vi "Plotter.vi"(1 "3rd":string[](array[string]), 2 "2nd":string[](array[string])) -> (0 "Desired Indicies":i32[](array[numeric]))   [LabVIEW 2010]
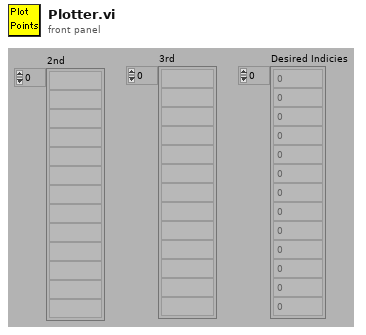
[diagram p1: front panel]
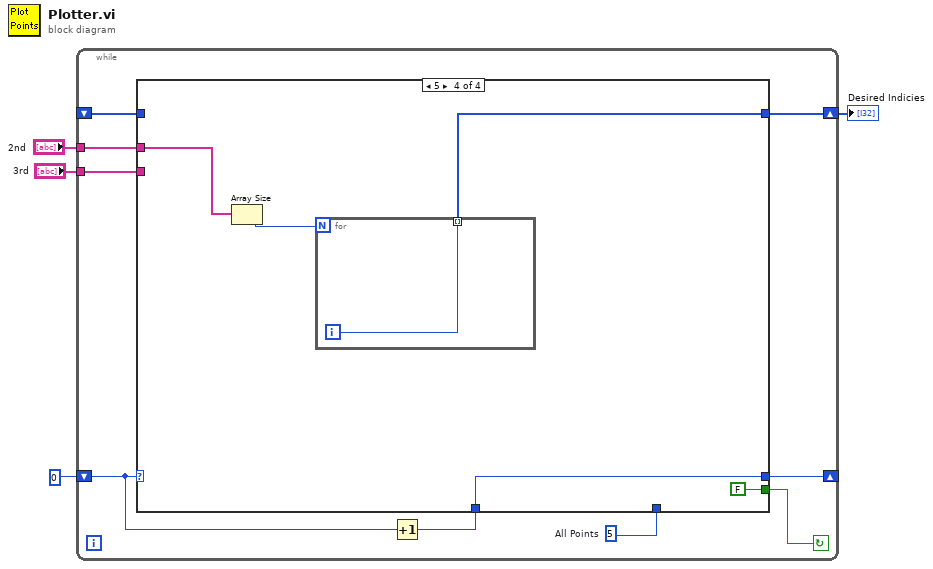
[diagram p0: block diagram]
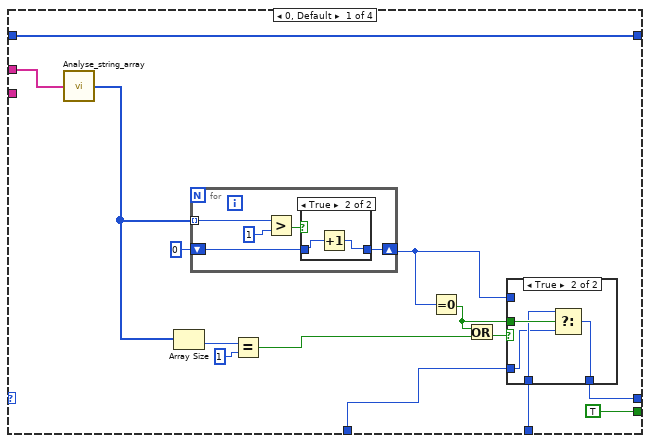
[diagram p2: hidden frame]
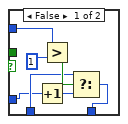
[diagram p3: hidden frame]
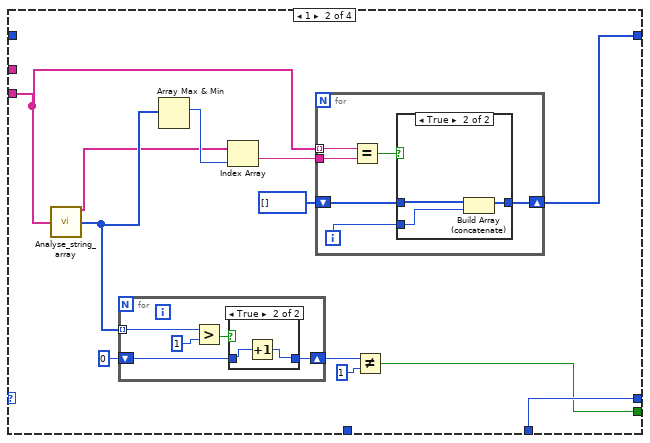
[diagram p5: hidden frame]
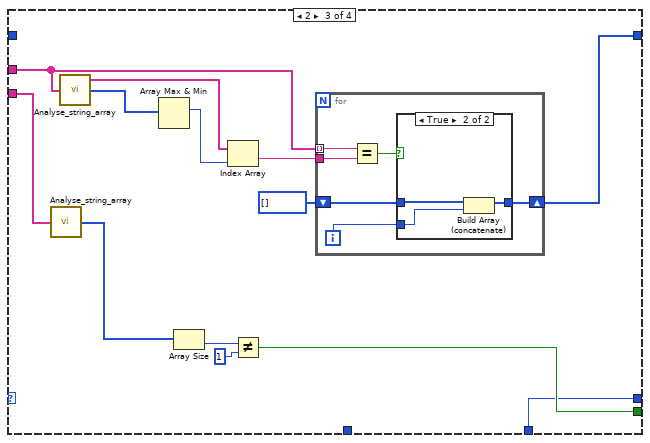
[diagram p8: hidden frame]
diagram:
  n1 = while {
    shift-left: _ -> [w5]
    shift-right: [w7] -> w1
    tunnel: "3rd" -> [w8]
    tunnel: "2nd" -> [w9]
    shift-left: 0 -> [w12]
    shift-right: [w10] -> _
    stop <- w13 continue-if-true
    w6 = 5  # All Points
    n2 = Increment(x=w12) -> (x+1=w11:i32)
    n3 = case shown="5" w12 {
      tunnel: [TRUE w50 w87 FALSE] -> w13
      tunnel: w11 -> [w18 _ _ w100]
      tunnel: [w19 w58 w86 w100] -> w10
      tunnel: w9 -> [w26 _ w79 w104]
      tunnel: w8 -> [_ w47 w80 _]
      tunnel: [w15 w54 w82 w102] -> w7
      tunnel: w6 -> [w16 w58 w86 _]
      tunnel: w5 -> [w15 _ _ _]
      frame 0, Default {
        n4 = call "Analyse_string_array.vi"("String array"=w26) -> ("Frequency"=w24:i32[])  [unwired: 1 in, 1 out]
        n5 = Array Size(array=w24) -> (size(s)=w22:i32)
        n6 = for {
          tunnel: w24 -> [w43] mode=indexing
          shift-right: [w40] -> w17
          shift-left: 0 -> [w39]
          n7 = Greater?(x=w43, y=1) -> (0:w41:bool)
          n8 = case shown="True" w41 {
            tunnel: [w44 w45] -> w40
            tunnel: w39 -> [w44 w46]
            frame False {
            }
            frame True {
              n9 = Increment(x=w46) -> (x+1=w45:i32)
            }
          }
        }
        n10 = Equal?(x=w22, y=1) -> (x = y?=w21:bool)
        n11 = Equal To 0?(x=w17) -> (x = 0?=w14:bool)
        n12 = Or(x=w14, y=w21) -> (x .or. y?=w20:bool)
        n13 = case shown="True" w20 {
          tunnel: [w28 w35] -> w19
          tunnel: w18 -> [w30 w36]
          tunnel: w17 -> [w34 _]
          tunnel: w16 -> [w31 w37]
          tunnel: w14 -> [_ w38]
          frame False {
            n14 = Increment(x=w30) -> (x+1=w29:i32)
            n15 = Greater?(x=w34, y=1) -> (0:w32:bool)
            n16 = Select(t=w31, s=w32, f=w29) -> (s? t:f=w28:i32)
          }
          frame True {
            n17 = Select(t=w37, s=w38, f=w36) -> (s? t:f=w35:i32)
          }
        }
      }
      frame 1 {
        n18 = call "Analyse_string_array.vi"("String array"=w47) -> ("Unique strings"=w48:string[], "Frequency"=w49:i32[])  [unwired: 1 in]
        n19 = for {
          tunnel: w49 -> [w63] mode=indexing
          shift-right: [w60] -> w51
          shift-left: 0 -> [w59]
          n20 = Greater?(x=w63, y=1) -> (0:w61:bool)
          n21 = case shown="True" w61 {
            tunnel: [w64 w65] -> w60
            tunnel: w59 -> [w64 w66]
            frame False {
            }
            frame True {
              n22 = Increment(x=w66) -> (x+1=w65:i32)
            }
          }
        }
        n23 = Array Max & Min(array=w49) -> (max index (indices)=w57:i32)  [unwired: 3 out]
        n24 = Index Array(array=w48, index=w57) -> (element=w56:string)
        n25 = for {
          shift-right: [w68] -> w54
          shift-left: i32[] [] -> [w69]
          tunnel: w47 -> [w72] mode=indexing
          tunnel: w56 -> [w71]
          i -> [w67]
          n26 = Equal?(x=w72, y=w71) -> (x = y?=w70:bool)
          n27 = case shown="True" w70 {
            tunnel: w69 -> [w73 w76]
            tunnel: [w73 w74] -> w68
            tunnel: w67 -> [_ w75]
            frame False {
            }
            frame True {
              n28 = Build Array (concatenate)(w76, w75) -> (w74:i32[])
            }
          }
        }
        n29 = Not Equal?(x=w51, y=1) -> (x != y?=w50:bool)
      }
      frame 2 {
        n30 = call "Analyse_string_array.vi"("String array"=w80) -> ("Frequency"=w81:i32[])  [unwired: 1 in, 1 out]
        n31 = call "Analyse_string_array.vi"("String array"=w79) -> ("Unique strings"=w77:string[], "Frequency"=w78:i32[])  [unwired: 1 in]
        n32 = Array Max & Min(array=w78) -> (max index (indices)=w85:i32)  [unwired: 3 out]
        n33 = Array Size(array=w81) -> (size(s)=w88:i32)
        n34 = Index Array(array=w77, index=w85) -> (element=w84:string)
        n35 = Not Equal?(x=w88, y=1) -> (x != y?=w87:bool)
        n36 = for {
          shift-right: [w91] -> w82
          shift-left: i32[] [] -> [w92]
          tunnel: w79 -> [w95] mode=indexing
          tunnel: w84 -> [w94]
          i -> [w90]
          n37 = Equal?(x=w95, y=w94) -> (x = y?=w93:bool)
          n38 = case shown="True" w93 {
            tunnel: w92 -> [w96 w99]
            tunnel: [w96 w97] -> w91
            tunnel: w90 -> [_ w98]
            frame False {
            }
            frame True {
              n39 = Build Array (concatenate)(w99, w98) -> (w97:i32[])
            }
          }
        }
      }
      frame 5 {
        n40 = Array Size(array=w104) -> (size(s)=w103:i32)
        n41 = for {
          N: w103 -> [_]
          tunnel: [w105] -> w102 mode=indexing
          i -> [w105]
        }
      }
    }
  }
  "Desired Indicies" <- w1
